vi "Right Motor Init.vi"(8 "error in":errorcluster, 10 "Invert (default false)":bool, 11 "CAN Id":u8) -> (0 "error out":errorcluster)   [LabVIEW 2014]
uses:
  Global Objects.vi
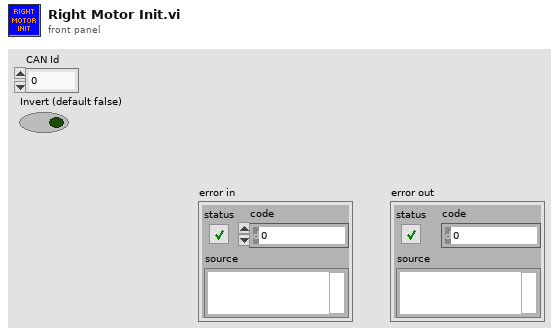
[diagram p1: front panel]
types:
  T1 = typedef "Motor Typedef.ctl" = cluster{"MotorControlDeviceRef":T2}
  T2 = typedef "WPI_MotorControlDeviceRef.ctl" = cluster{"DeviceStatus":errorcluster, "Type":T3, "PWM":cluster{"Controller":T4, "PWM Channel":T5, "DeadBand":T6}, "CAN":cluster{"Device Number":u8, "Control Mode":T7, "Semaphore":T8, "Max Vout":dbl, "TalonSRX Control Mode":T9}, "Invert":bool, "TransformRef":T10, "InvTransformRef":T10}
  T3 = typedef "WPI_MotorControlType.ctl" = enum16{"PWM", "CAN", "CANTalonSRX"}
  T4 = typedef "FPGA_TypedefDigitalModule.ctl" = enum16{"Controller 1"}
  T5 = typedef "FPGA_DIOPWMChannel.ctl" = enum8{"PWM 0", "PWM 1", "PWM 2", "PWM 3", "PWM 4", "PWM 5", "PWM 6", "PWM 7", "PWM 8", "PWM 9", "PWM MXP 0", "PWM MXP 1", "PWM MXP 2", "PWM MXP 3", "PWM MXP 4", "PWM MXP 5", "PWM MXP 6", "PWM MXP 7", "PWM MXP 8", "PWM MXP 9", "Invalid"}
  T6 = typedef "WPI_PWMDeadband.ctl" = cluster{"Name":string, "maxPositivePwm":i32, "minPositivePwm":i32, "centerPwm":i32, "maxNegativePwm":i32, "minNegativePwm":i32, "angularRange":u16}
  T7 = typedef "WPI_CANJaguar_ControlMode.ctl" = enum8{"Percent VBus", "Current", "Speed", "Position", "Voltage"}
  T8 = typedef "Semaphore RefNum" = refnum<k1>
  T9 = typedef "WPI_CANTalonSRX_APIControlMode.ctl" = enum8{"Percent VBus", "Speed", "Position", "Slave", "Unchanged / Invalid"}
  T10 = typedef "WPI_PWMTransform_ConPane.ctl" = refnum<vi>
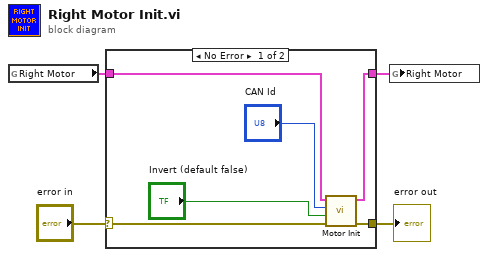
[diagram p0: block diagram]
diagram:
  n1 = global read "Global Objects.vi" "Right Motor"() -> (w2:T1)
  n2 = case shown="No Error" "error in" {
    selector: "error in" -> [w8 w12]
    tunnel: [w7 w12] -> w3
    tunnel: w2 -> [w10 w11]
    tunnel: [w9 w11] -> w1
    frame No Error {
      n3 = call "Motor Init.vi"("error in"=w8, "Invert (default false)"="Invert (default false)", "CAN Id"="CAN Id", "Motor In"=w10) -> ("error out"=w7:errorcluster, "Motor Out"=w9:T1)  [unwired: 6 in]
    }
    frame Error {
    }
  }
  "error out" <- w3
  n4 = global write "Global Objects.vi" "Right Motor"(w1) -> ()
